vi "Panel.vi"(11 "TipTablePanel in":refnum<class "TipTablePanel.lvclass">) -> ()   [LabVIEW 2021, in "RocketPlot.lvlib" / "TipTablePanel.lvclass"]
uses:
  TipTablePanel.lvclass
  C:/Program Files/National Instruments/LabVIEW 2021/user.lib/bjustice/TipStripOOPanel/Classes/TipPanel/TipPanel.lvclass
  C:/Program Files/National Instruments/LabVIEW 2021/vi.lib/IlluminatedG/IG OOPanel/OOPanel/Panel/Panel.lvclass
  <vilib>/Utility/miscctls.llb/LVPositionTypeDef.ctl
  <vilib>/Utility/miscctls.llb/LVRowAndColumnTypeDef.ctl
  <userlib>/bjustice/TipStripOOPanel/Classes/TipPanel/TipPanel.lvclass/TipPanel.ctl
  TipTablePanel.lvclass/TipTablePanel.ctl
  <userlib>/bjustice/TipStripOOPanel/Classes/TipPanel/Read New Panel UE.vi
  <vilib>/Futures/Futures/Promise/Promise.lvclass
  <vilib>/IlluminatedG/IG OOPanel/OOPanel/Panel/Panel.lvclass
  <vilib>/IlluminatedG/IG OOPanel/OOPanel/OOPanel.lvlib
  <userlib>/bjustice/TipStripOOPanel/Classes/TipPanel/TipPanel.lvclass
panel:
  out "Table Control":string[][](table)
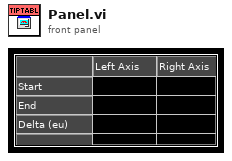
[diagram p1: front panel]
types:
  T1 = typedef "LVRowAndColumnTypeDef.ctl" = cluster{"Row":i32, "Column":i32}
  T2 = typedef "LVPositionTypeDef.ctl" = cluster{"Left":i32, "Top":i32}
  T3 = typedef "OOPanel.lvlib/Panel.lvclass/Panel Events.ctl" = cluster{"Visbility":refnum<user-event>, "Close":refnum<user-event>}
  T4 = typedef "OOPanel.lvlib/Visibility State.ctl" = enum16{"Idle", "Closed", "Hidden", "Visible", "Subpanel", "Hidden Subpanel"}
  T5 = typedef "TipStrip2.lvlib/TipPanel.lvclass/ToPanelUE.ctl" = cluster{"TipPanel":refnum<class>, "Promise.Size":refnum<class "Promise.lvclass">}
  T6 = typedef "RocketPlot.lvlib/TipTablePanel.lvclass/new tip instructions.ctl" = cluster{"Row Headers":string[], "Column Headers":string[], "cells":T7[][], "color":T8}
  T7 = typedef "RocketPlot.lvlib/TipTablePanel.lvclass/cell cache.ctl" = cluster{"text":string, "Color":u32, "Justification":enum16{"Left", "Center", "Right"}}
  T8 = typedef "RocketPlot.lvlib/TipTablePanel.lvclass/colors.ctl" = cluster{"Cell BG color":u32, "Cell font color":u32, "Row Header BG color":u32, "Row Header font color":u32, "Column Header BG color":u32, "Column Header font color":u32}
  T9 = typedef "LVBoundsTypeDef.ctl" = cluster{"Width":u32, "Height":u32}
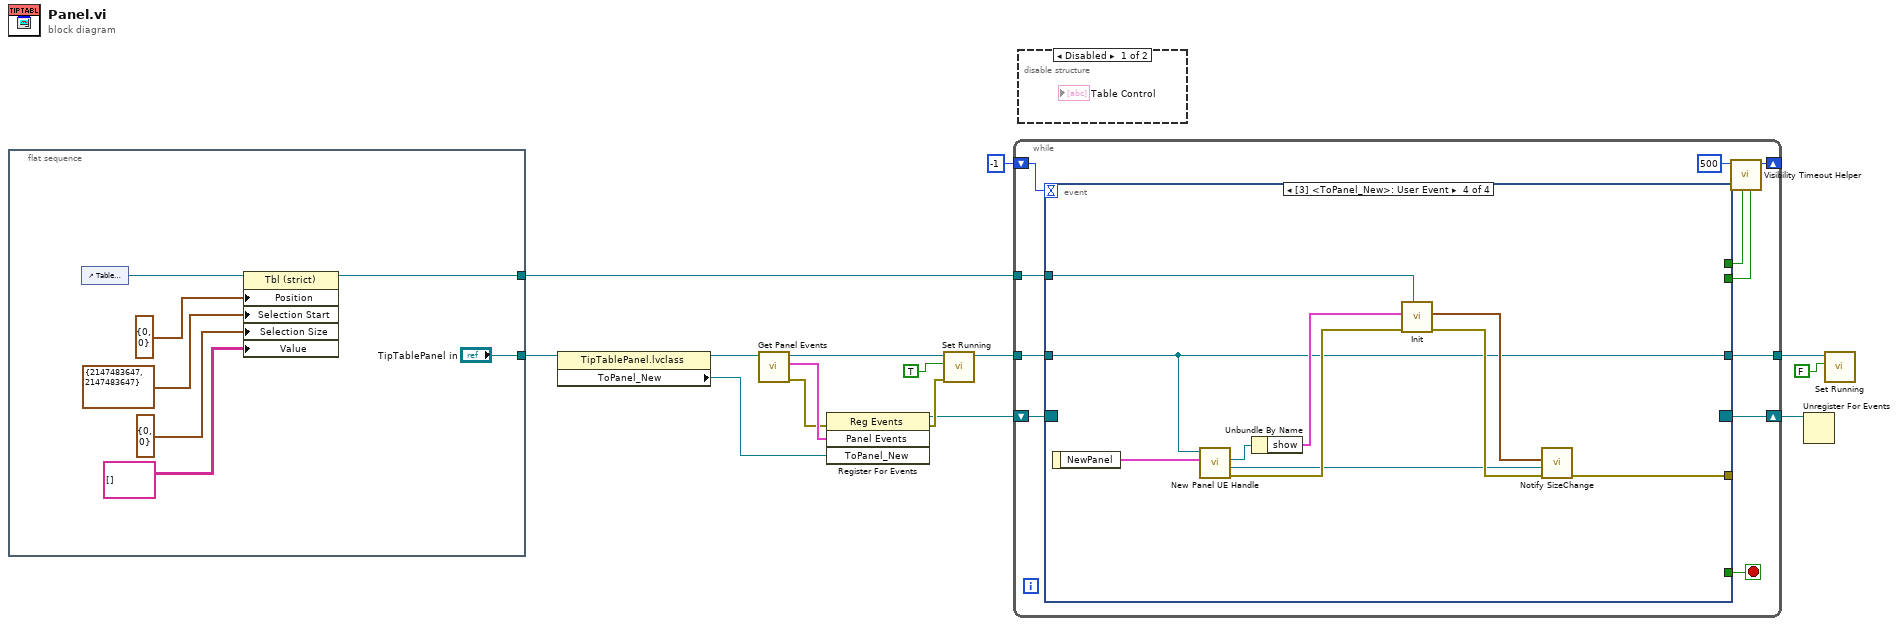
[diagram p0: block diagram]
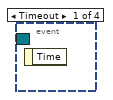
[diagram p3: hidden frame]
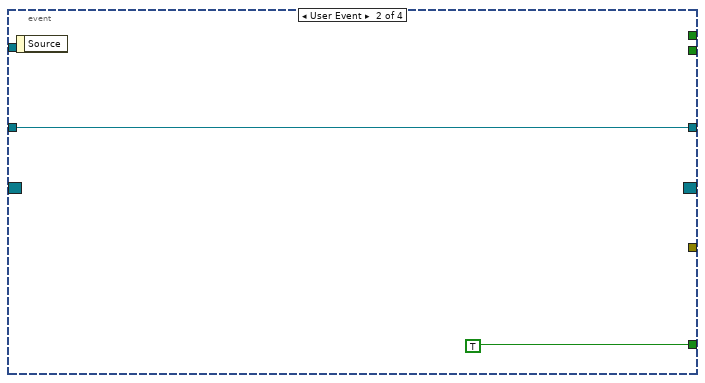
[diagram p4: hidden frame]
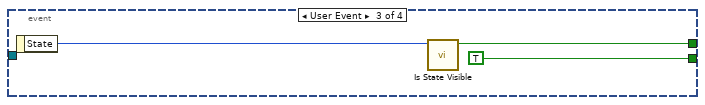
[diagram p5: hidden frame]
diagram:
  n1 = flat-sequence {
    tunnel: ["TipTablePanel in"] -> w4
    tunnel: [w16] -> w1
    frame #0 {
      n2 = control-ref of="Table Control"() -> (w18:refnum<vi>)
      n3 = property class="Tbl (strict)"(reference=w18, "Position"=T2 {"Left"=0, "Top"=0}, "Selection Start"=T1 {"Row"=2147483647, "Column"=2147483647}, "Selection Size"=T1 {"Row"=0, "Column"=0}, "Value"=string[][] [] ("Table Control")) -> (reference out=w16:refnum<vi>)  [unwired: 1 in, 1 out]
    }
  }
  n4 = property class="TipTablePanel.lvclass"(reference=w4) -> (reference out=w2:refnum<class "TipTablePanel.lvclass">, "ToPanel_New"=w3:refnum<user-event>)  [unwired: 1 in, 1 out]
  n5 = call <vilib>:"Get Panel Events.vi"("Panel in"=w2) -> ("error out"=w5:errorcluster, "Panel Events"=w15:T3, "Panel out"=w14:refnum<class "TipTablePanel.lvclass">)  [unwired: 8 in]
  n6 = register-events(error in=w5, w15, w3) -> (reference out=w11:refnum<event-registration>, error out=w12:errorcluster)  [unwired: 1 in]
  n7 = call <vilib>:"Set Running.vi"("error in (no error)"=w12, "Running"=TRUE, "Panel in"=w14) -> ("Panel out"=w10:refnum<class "TipTablePanel.lvclass">)  [unwired: 7 in, 1 out]
  n8 = while {
    shift-right: [w29] -> w7
    shift-left: w11 -> [w30]
    shift-right: [w32] -> _
    shift-left: -1 ("Timeout") -> [w31]
    tunnel: w10 -> [w25]
    tunnel: [w24] -> w6
    tunnel: w1 -> [w23]
    stop <- w26 stop-if-true
    n9 = event shown="[3] <ToPanel_New>: User Event" {
      selector: w30 -> [_ _ _ _]
      dyn-events: [_ _ _ _] -> w29
      timeout: w31 -> [_ _ _ _]
      tunnel: [_ _ w37 _] -> w28
      tunnel: [_ _ TRUE _] -> w27
      tunnel: [_ TRUE _ _] -> w26
      tunnel: w25 -> [_ w34 _ w41]
      tunnel: [_ w34 _ w41] -> w24
      tunnel: w23 -> [_ _ _ w47]
      tunnel: [_ _ _ w42] -> _
      event Timeout {
        n10 = event-data() -> ()  [unwired: 1 in, 1 out]
      }
      event User Event {
        n11 = event-data() -> ()  [unwired: 1 in, 1 out]
      }
      event User Event {
        n12 = event-data() -> ("State"=w38:T4)  [unwired: 1 in]
        n13 = call <vilib>:"Is State Visible.vi"("Visibility"=w38) -> ("Visible"=w37:bool)  [unwired: 10 in]
      }
      event User Event {
        n14 = event-data() -> ("NewPanel"=w48:T5)  [unwired: 1 in]
        n15 = call <userlib>:"New Panel UE Handle.vi"("NewPanel"=w48, "TipPanel in"=w41) -> ("error out"=w43:errorcluster, "Promise.Size"=w39:refnum<class "Promise.lvclass">, "DATA ONLY"=w40:refnum<class "TipTablePanel.lvclass">)  [unwired: 7 in]
        n16 = Unbundle By Name(w40) -> ("show"=w44:T6)
        n17 = call "Init.vi"("TableRef"=w47, "error in (no error)"=w43, "show"=w44) -> ("error out"=w45:errorcluster, "Size"=w46:T9)  [unwired: 7 in]
        n18 = call <userlib>:"Notify SizeChange.vi"("error in (no error)"=w45, "Promise in"=w39, "content size"=w46) -> ("error out"=w42:errorcluster)  [unwired: 8 in]
      }
    }
    n19 = call <vilib>:"Visibility Timeout Helper.vi"("Update?"=w27, "Use Timeout?"=w28, "Visible Timeout mS"=500) -> ("Timeout"=w32:i32)  [unwired: 8 in]
  }
  n20 = disable-structure shown="Disabled" {
    frame Disabled {
    }
    frame Enabled {
    }
  }
  n21 = Unregister For Events(event registration refnum=w7) -> ()  [unwired: 1 in, 1 out]
  n22 = call <vilib>:"Set Running.vi"("Running"=FALSE, "Panel in"=w6) -> ()  [unwired: 8 in, 2 out]
